vi "Check If Line Exists.vi"(8 "error in":errorcluster, 10 "Name to Locate":string, 11 "JSON_RPC_Interface configuration in":refnum<class "JSON_RPC_Interface configuration.lvclass">) -> (0 "error out":errorcluster, 1 "Index":i32, 2 "Line out":T1, 3 "JSON_RPC_Interface configuration out":refnum<class "JSON_RPC_Interface configuration.lvclass">, 5 "Found?":bool)   [LabVIEW 2017, in "JSON_RPC_Interface configuration.lvclass"]
doc: "Checks if a line already exists within a configuration."
uses:
  JSON_RPC_Interface configuration.lvclass
  Line.ctl
  <vilib>/NI/Tag Bus Module Framework/channel/TBM channel.lvclass
  JSON_RPC_Interface configuration.lvclass/JSON_RPC_Interface configuration.ctl
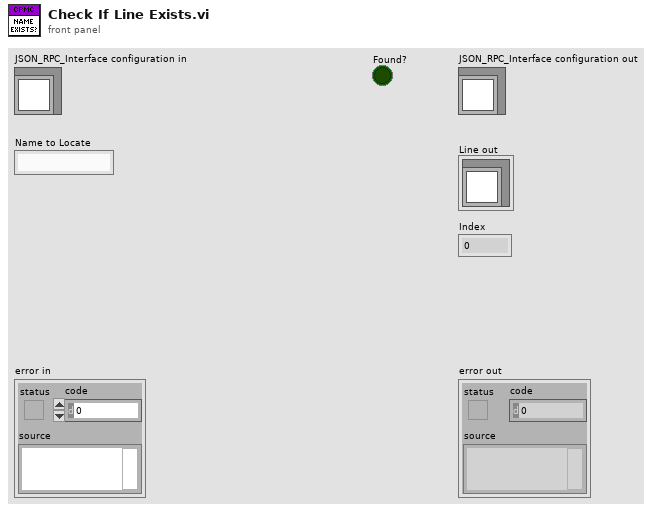
[diagram p1: front panel]
types:
  T1 = typedef "JSON_RPC_Interface configuration.lvclass/Line.ctl" = cluster{"channel":refnum<class "TBM channel.lvclass">}
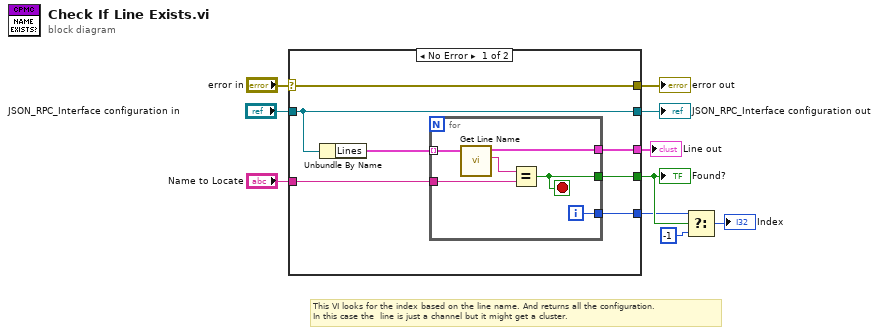
[diagram p0: block diagram]
diagram:
  # "This VI looks for the index based on the line name. And returns all the configuration. \nIn this case the  line is just a channel but it might get a cluster."
  n1 = case shown="No Error" "error in" {
    selector: "error in" -> [w17 w25]
    tunnel: [w17 w25] -> w9
    tunnel: [w16 w24] -> w7
    tunnel: "JSON_RPC_Interface configuration in" -> [w16 w24]
    tunnel: "Name to Locate" -> [w14 _]
    tunnel: [w13 _] -> w3
    tunnel: [w12 _] -> w2
    tunnel: [w11 _] -> w1
    frame No Error {
      n2 = Unbundle By Name(w16) -> ("Lines"=w15:T1[])
      n3 = for {
        tunnel: w15 -> [w18] mode=indexing
        tunnel: w14 -> [w23]
        tunnel: [w22] -> w13
        tunnel: [w21] -> w12
        tunnel: [w19] -> w11
        i -> [w21]
        stop <- w22 stop-if-true
        n4 = call "Get Line Name.vi"("Line in"=w18) -> ("Name"=w20:string, "Line out"=w19:T1)  [unwired: 8 in, 1 out]
        n5 = Equal?(x=w20, y=w23) -> (x = y?=w22:bool)
      }
    }
    frame Error {
    }
  }
  "error out" <- w9
  "JSON_RPC_Interface configuration out" <- w7
  "Found?" <- w3
  "Line out" <- w1
  n6 = Select(t=w2, s=w3, f=-1) -> (s? t:f=→"Index":i32)
